vi "labo01.01.vi"() -> ()   [LabVIEW 2020]
panel:
  out "done":string
  in  "try 2":string
  in  "try 01":string
  out "Zdanie stwrzone z podanych s丑w:":string
  in  "Slowo  8:":string
  in  "Slowo  7:":string
  in  "Slowo  6:":string
  in  "Slowo  5:":string
  in  "Slowo  4:":string
  in  "Slowo  3:":string
  in  "Slowo  2:":string
  in  "Slowo 1:":string
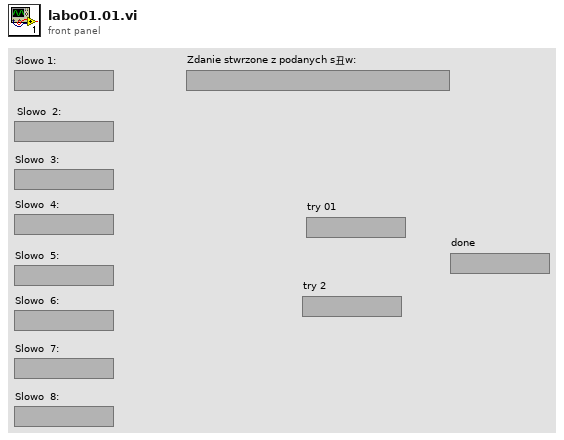
[diagram p1: front panel]
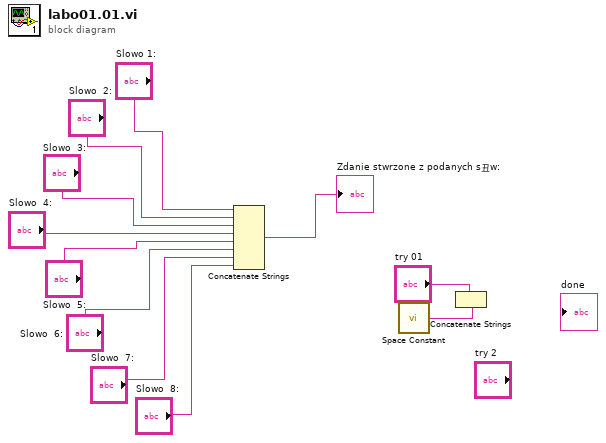
[diagram p0: block diagram]
diagram:
  n1 = Concatenate Strings("Slowo 1:", "Slowo  2:", "Slowo  3:", "Slowo  4:", "Slowo  5:", "Slowo  6:", "Slowo  7:", "Slowo  8:") -> (→"Zdanie stwrzone z podanych s丑w:":string)
  n2 = call <vilib>:"Space Constant.vi"() -> ("String"=w2:string)
  n3 = Concatenate Strings("try 01", w2) -> ()  [unwired: 1 out]
